vi "Format Unique Output File Name.vi"(0 "current dir":path, 5 "target dir":path, 11 "error in":errorcluster) -> (4 "output file name":string, 6 "root file":bool, 8 "header string":string, 15 "error out":errorcluster)   [LabVIEW 2019, in "MD Generator.lvlib"]
doc: "This VI checks the current directory against target directory, and builds output file name approiately.\nIf target and current are equal, then make name \"VI Reference\"."
uses:
  MD Generator.lvlib
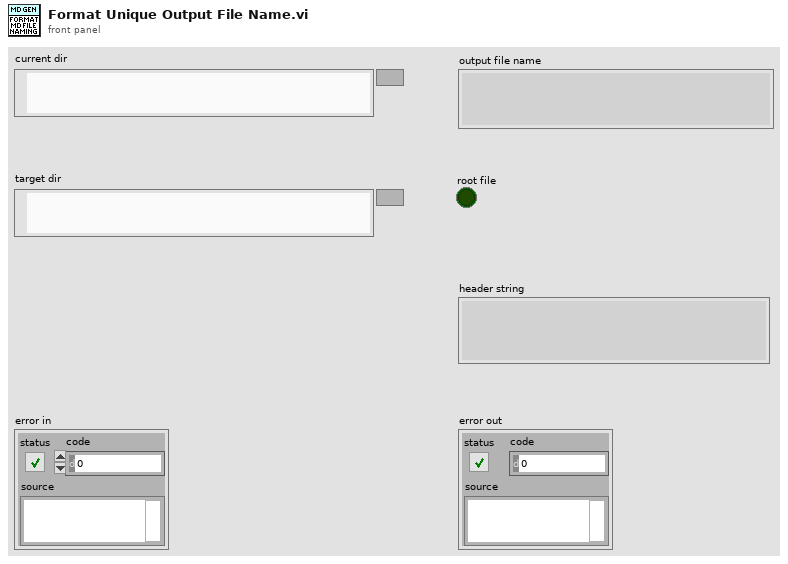
[diagram p1: front panel]
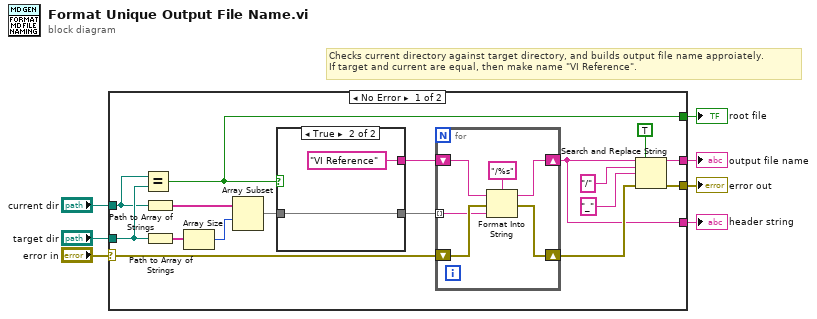
[diagram p0: block diagram]
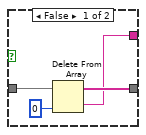
[diagram p2: hidden frame]
diagram:
  # "Checks current directory against target directory, and builds output file name approiately.\nIf target and current are equal, then make name \"VI Reference\"."
  n1 = case shown="No Error" "error in" {
    selector: "error in" -> [w24 w37]
    tunnel: [w22 w37] -> w6
    tunnel: [w21 _] -> w5
    tunnel: "target dir" -> [w16 _]
    tunnel: "current dir" -> [w15 _]
    tunnel: [w11 _] -> w2
    tunnel: [w8 _] -> w1
    frame No Error {
      n2 = Equal?(x=w15, y=w16) -> (x = y?=w11:bool)
      n3 = Path to Array of Strings(0:w15) -> (2:w19:string[])  [unwired: 1 out]
      n4 = Path to Array of Strings(0:w16) -> (2:w18:string[])  [unwired: 1 out]
      n5 = Array Size(array=w18) -> (size(s)=w14:i32)
      n6 = Array Subset(array=w19, index=w14) -> (w17:string[])  [unwired: 1 in]
      n7 = case shown="True" w11 {
        tunnel: w17 -> [w28 w29]
        tunnel: [w27 w29] -> w13
        tunnel: [w26 "VI Reference"] -> w12
        frame False {
          n8 = Delete From Array(array=w28, index=0) -> (deleted portion=w26:string, array with subset deleted=w27:string[])  [unwired: 1 in]
        }
        frame True {
        }
      }
      n9 = for {
        shift-right: [w35] -> w10
        shift-left: w24 -> [w34]
        shift-right: [w36] -> w8
        shift-left: w12 -> [w33]
        tunnel: w13 -> [w31] mode=indexing
        n10 = Format Into String(format string="/%s", initial string=w33, error in=w34, w31) -> (resulting string=w36:string, error out=w35:errorcluster)
      }
      n11 = Search and Replace String(replace all?=TRUE ("replace all? (F)"), input string=w8, search string="/", replace string="_" ("replace string (\"\")"), error in=w10) -> (result string=w21:string, error out=w22:errorcluster)  [unwired: 3 in, 2 out]
    }
    frame Error {
    }
  }
  "error out" <- w6
  "output file name" <- w5
  "root file" <- w2
  "header string" <- w1
